vi "Create Slice.vi"(6 "Draw Mode":T1(ring)=enum."Triangles", 7 "3D Pie Property":T5, 8 "error in (no error)":errorcluster, 10 "Plot Representation In":T2, 11 "Plot Object In":refnum<vi>) -> (0 "error out":errorcluster, 2 "Plot Representation Out":T2, 3 "Plot Object Out":refnum<vi>, 4 "Sector Object Out":refnum<vi>, 5 "Drawable":refnum<vi>)   [LabVIEW 2017, in "3D Pie.lvclass"]
uses:
  <vilib>/Math Plots/3D Math Plots/3D Pie/3D Pie/3D Pie.lvclass
  <vilib>/Math Plots/3D Math Plots/3D Pie/3D Pie/Typedef/3D Pie Property.ctl
  <vilib>/Math Plots/3D Math Plots/3D Plot/3D Plot/Typedef/Line Type.ctl
  <vilib>/Math Plots/3D Math Plots/3D Plot/3D Plot/Typedef/Plot Representation.ctl
  <vilib>/Math Plots/3D Math Plots/3D Plot/3D Plot/Typedef/Range Clusters.ctl
  <vilib>/Math Plots/3D Math Plots/3D Plot/3D Plot/Typedef/Mesh Data.ctl
  <vilib>/picture/3D Picture Control/NI_3D Picture Control.lvlib
  <vilib>/Math Plots/3D Math Plots/3D Plot/3D Plot/3D Plot.lvclass
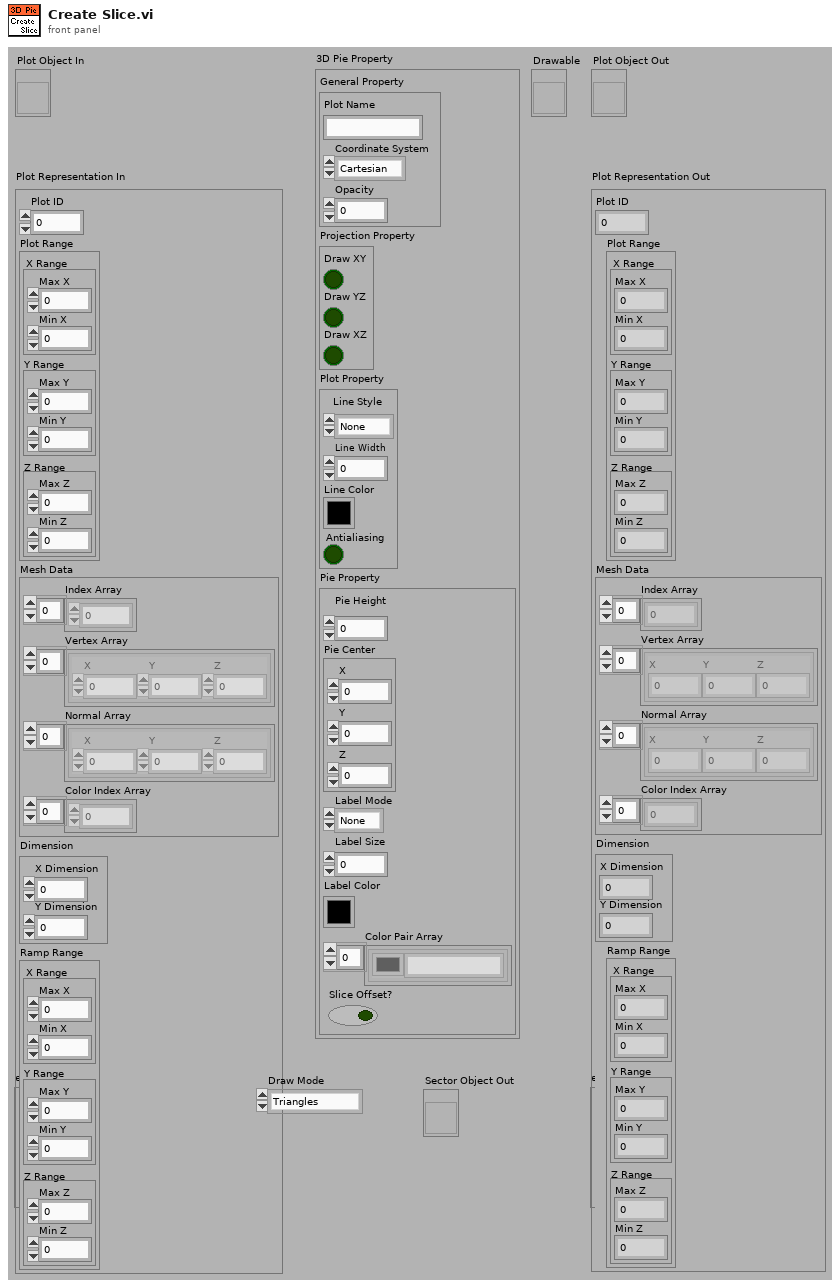
[diagram p1: front panel]
types:
  T1 = enum16{"Points", "Lines", "Line Strip", "Line Loop", "Triangles", "Triangle Strip", "Triangle Fan", "Quads", "Quad Strip", "Polygon"}
  T2 = typedef "3D Plot.lvclass/Plot Representation.ctl" = cluster{"Plot ID":i32, "Plot Range":T3, "Mesh Data":T4, "Dimension":cluster{"X Dimension":i32, "Y Dimension":i32}, "Ramp Range":T3}
  T3 = typedef "3D Plot.lvclass/Range Clusters.ctl" = cluster{"X Range":cluster{"Max X":sgl, "Min X":sgl}, "Y Range":cluster{"Max Y":sgl, "Min Y":sgl}, "Z Range":cluster{"Max Z":sgl, "Min Z":sgl}}
  T4 = typedef "3D Plot.lvclass/Mesh Data.ctl" = cluster{"Index Array":u32[], "Vertex Array":cluster{"X":sgl, "Y":sgl, "Z":sgl}[], "Normal Array":cluster{"X":sgl, "Y":sgl, "Z":sgl}[], "Color Index Array":i32[]}
  T5 = typedef "3D Pie.lvclass/3D Pie Property.ctl" = cluster{"General Property":cluster{"Plot Name":string, "Coordinate System":enum16{"Cartesian", "Cylindrical", "Spherical"}, "Opacity":sgl}, "Projection Property":cluster{"Draw XY":bool, "Draw YZ":bool, "Draw XZ":bool}, "Plot Property":cluster{"Line Style":T6, "Line Width":sgl, "Line Color":u32, "Antialiasing":bool}, "Pie Property":cluster{"Pie Height":sgl, "Pie Center":cluster{"X":sgl, "Y":sgl, "Z":sgl}, "Label Mode":enum16{"None", "Show Percentage", "Show String"}, "Label Size":u16, "Label Color":u32, "Color Pair Array":cluster{"Color":u32, "String":string}[], "Slice Offset?":bool}}
  T6 = typedef "3D Plot.lvclass/Line Type.ctl" = enum16{"None", "Solid", "Dash", "Dot", "Dash Dot"}
  T7 = enum16{"Overall", "Per Primitive", "Per Vertex", "Binding Off"}
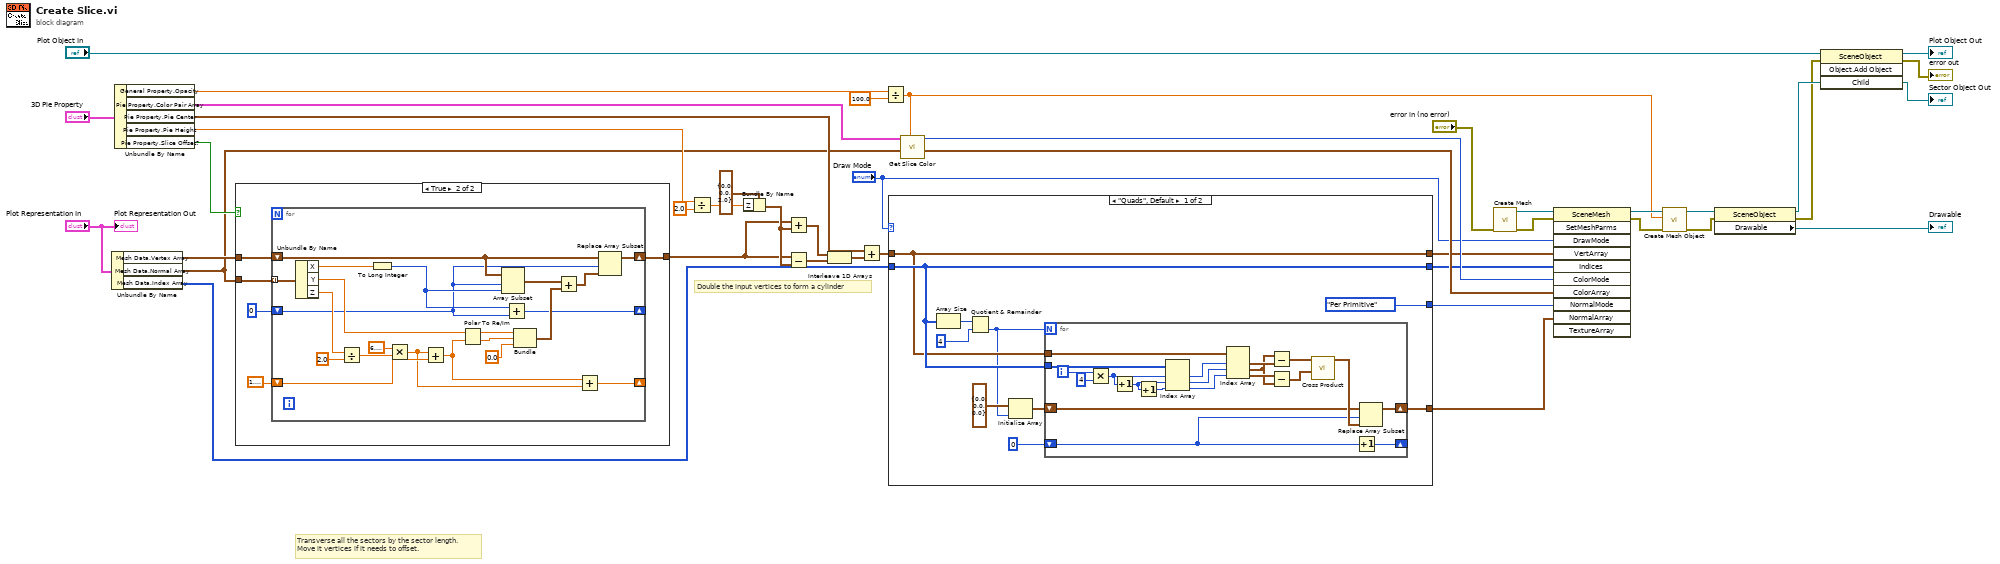
[diagram p0: block diagram]
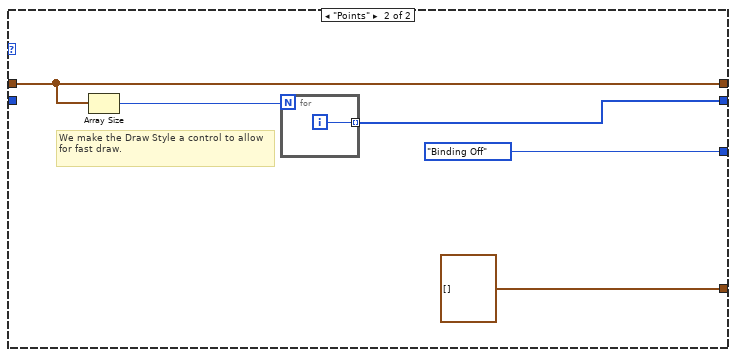
[diagram p2: hidden frame]
diagram:
  # "Double the input vertices to form a cylinder"
  # "Transverse all the sectors by the sector length.\nMove it vertices if it needs to offset."
  n1 = Unbundle By Name("Plot Representation In") -> ("Mesh Data.Vertex Array"=w27:cluster{"X":sgl, "Y":sgl, "Z":sgl}[], "Mesh Data.Normal Array"=w10:cluster{"X":sgl, "Y":sgl, "Z":sgl}[], "Mesh Data.Index Array"=w7:u32[])
  n2 = Unbundle By Name("3D Pie Property") -> ("General Property.Opacity"=w15:sgl, "Pie Property.Color Pair Array"=w9:cluster{"Color":u32, "String":string}[], "Pie Property.Pie Center"=w20:cluster{"X":sgl, "Y":sgl, "Z":sgl}, "Pie Property.Pie Height"=w21:sgl, "Pie Property.Slice Offset?"=w25:bool)
  n3 = case shown="True" w25 {
    tunnel: w10 -> [_ w48]
    tunnel: w27 -> [w43 w47]
    tunnel: [w43 w46] -> w26
    frame False {
    }
    frame True {
      n4 = for {
        tunnel: w48 -> [w70] mode=indexing
        shift-right: [w49] -> w46
        shift-left: w47 -> [w52]
        shift-right: [w60] -> _
        shift-left: 0 ("index") -> [w51]
        shift-right: [w63] -> _
        shift-left: sgl 1.5707964 -> [w62]
        n5 = Unbundle By Name(w70) -> ("X"=w69:sgl, "Y"=w68:sgl, "Z"=w65:sgl)
        n6 = Divide(x=w65, y=sgl 2.0) -> (x/y=w57:sgl)
        n7 = To Long Integer(number=w69) -> (32bit integer=w54:i32)
        n8 = Multiply(x=sgl 6.2831855, y=w57) -> (x*y=w55:sgl)
        n9 = Add(x=w55, y=w62) -> (x+y=w56:sgl)
        n10 = Polar To Re/Im(2:w56, 3:w68) -> (0:w58:sgl, 1:w59:sgl)
        n11 = Array Subset(array=w52, index=w51, length=w54) -> (w53:cluster{"X":sgl, "Y":sgl, "Z":sgl}[])
        n12 = Add(x=w54, y=w51) -> (x+y=w60:i32)
        n13 = Bundle(w59, w58, "y"=sgl 0.0) -> (w66:cluster{sgl, sgl, "y":sgl})  [unwired: 1 out]
        n14 = Add(x=w53, y=w66) -> (x+y=w50:cluster{sgl, sgl, sgl}[])
        n15 = Add(x=w56, y=w55) -> (x+y=w63:sgl)
        n16 = Replace Array Subset(array=w52, new element=w50, index=w51) -> (w49:cluster{"X":sgl, "Y":sgl, "Z":sgl}[])
      }
    }
  }
  n17 = Divide(x=w21, y=sgl 2.0) -> (x/y=w30:sgl)
  n18 = Bundle By Name(cluster=cluster{"X":sgl, "Y":sgl, "Z":sgl} {"X"=0.0, "Y"=0.0, "Z"=2.0} ("3D Point"), "Z"=w30) -> (w28:cluster{"X":sgl, "Y":sgl, "Z":sgl})
  n19 = Add(x=w26, y=w28) -> (x+y=w34:cluster{"X":sgl, "Y":sgl, "Z":sgl}[])
  n20 = Subtract(x=w26, y=w28) -> (x-y=w33:cluster{"X":sgl, "Y":sgl, "Z":sgl}[])
  n21 = Interleave 1D Arrays(w34, w33) -> (w22:cluster{"X":sgl, "Y":sgl, "Z":sgl}[])
  n22 = Add(x=w20, y=w22) -> (x+y=w18:cluster{"X":sgl, "Y":sgl, "Z":sgl}[])
  n23 = Divide(x=w15, y=sgl 100.0) -> (x/y=w8:sgl)
  n24 = case shown="\"Quads\", Default" "Draw Mode" {
    tunnel: w18 -> [w75 w104]
    tunnel: [w75 w104] -> w17
    tunnel: [w76 w103] -> w16
    tunnel: w7 -> [w76 _]
    tunnel: [T7."Per Primitive" ("Normal Binding Mode") T7."Binding Off" ("Normal Binding Mode")] -> w6
    tunnel: [w74 cluster{"X":sgl, "Y":sgl, "Z":sgl}[] [] ("Normal Array")] -> w5
    frame "Quads", Default {
      n25 = Array Size(array=w76) -> (size(s)=w79:i32)
      n26 = Quotient & Remainder(x=w79, y=4) -> (floor(x/y)=w72:i32)  [unwired: 1 out]
      n27 = Initialize Array(cluster{"X":sgl, "Y":sgl, "Z":sgl} {"X"=0.0, "Y"=0.0, "Z"=0.0} ("3D Point"), w72) -> (w77:cluster{"X":sgl, "Y":sgl, "Z":sgl}[])
      n28 = for {
        N: w72 -> [_]
        shift-right: [w87] -> w74
        shift-left: w77 -> [w88]
        tunnel: w76 -> [w98]
        tunnel: w75 -> [w97]
        shift-right: [w86] -> _
        shift-left: 0 -> [w85]
        i -> [w100]
        n29 = Multiply(x=w100, y=4) -> (x*y=w84:i32)
        n30 = Increment(x=w84) -> (x+1=w83:i32)
        n31 = Increment(x=w83) -> (x+1=w82:i32)
        n32 = Index Array(array=w98, index #1=w84, index #2=w83, index #3=w82) -> (element #1=w92:u32, element #2=w91:u32, element #3=w90:u32)
        n33 = Index Array(array=w97, index #1=w92, index #2=w91, index #3=w90) -> (element #1=w96:cluster{"X":sgl, "Y":sgl, "Z":sgl}, element #2=w81:cluster{"X":sgl, "Y":sgl, "Z":sgl}, element #3=w95:cluster{"X":sgl, "Y":sgl, "Z":sgl})
        n34 = Subtract(x=w81, y=w96) -> (x-y=w94:cluster{"X":sgl, "Y":sgl, "Z":sgl})
        n35 = Subtract(x=w95, y=w81) -> (x-y=w93:cluster{"X":sgl, "Y":sgl, "Z":sgl})
        n36 = call <vilib>:"Cross Product.vi"("Vector 2"=w93, "Vector 1"=w94) -> ("Vector Out"=w89:cluster{"X":sgl, "Y":sgl, "Z":sgl})  [unwired: 9 out]
        n37 = Increment(x=w85) -> (x+1=w86:i32)
        n38 = Replace Array Subset(array=w88, new element=w89, index=w85) -> (w87:cluster{"X":sgl, "Y":sgl, "Z":sgl}[])
      }
    }
    frame "Points" {
      # "We make the Draw Style a control to allow for fast draw."
      n39 = Array Size(array=w104) -> (size(s)=w105:i32)
      n40 = for {
        N: w105 -> [_]
        tunnel: [w106] -> w103 mode=indexing
        i -> [w106]
      }
    }
  }
  n41 = call <vilib>:"Get Slice Color.vi"("Opacity"=w8, "Normal Array"=w10, "Color Pair Array"=w9) -> ("Color Array"=w24:cluster{"R":sgl, "G":sgl, "B":sgl, "A":sgl}[], "Color Binding Mode"=w23:T7)  [unwired: 1 in, 6 out]
  n42 = call <vilib>:"Create Mesh.vi"("error in (no error)"="error in (no error)") -> ("error out"=w41:errorcluster, "New Mesh Refnum"=w42:refnum<vi>)  [unwired: 9 out]
  n43 = invoke class="SceneMesh" method="SetMeshParms"(reference=w42, error in=w41, "DrawMode"="Draw Mode", "VertArray"=w17, "Indices"=w16, "ColorMode"=w23, "ColorArray"=w24, "NormalMode"=w6, "NormalArray"=w5) -> (reference out=w13:refnum<vi>, error out=w14:errorcluster)  [unwired: 2 in, 9 out]
  n44 = call <vilib>:"Create Mesh Object.vi"("error in (no error)"=w14, "Alpha"=w8, "Mesh Object In"=w13) -> ("error out"=w2:errorcluster, "Object Ref Out"=w12:refnum<vi>)  [unwired: 1 in, 6 out]
  n45 = property class="SceneObject"(reference=w12, error in=w2) -> (reference out=w4:refnum<vi>, error out=w1:errorcluster, "Drawable"=→"Drawable":refnum<vi>)
  n46 = invoke class="SceneObject" method="Object.Add Object"(reference="Plot Object In", error in=w1, "Child"=w4) -> (reference out=→"Plot Object Out":refnum<vi>, error out=→"error out":errorcluster, "Child"=→"Sector Object Out":refnum<vi>)  [unwired: 1 in, 1 out]
  "Plot Representation Out" <- "Plot Representation In"
